vi "7HP_Get_serial_number.vi"(3 "timeout (ms)":u32=5000, 5 "Port":refnum<visa-resource-name>) -> (0 "Error Out":errorcluster, 2 "Serial number":u32)   [LabVIEW 2020]
uses:
  ctls/7HP_Cmd (USB).ctl
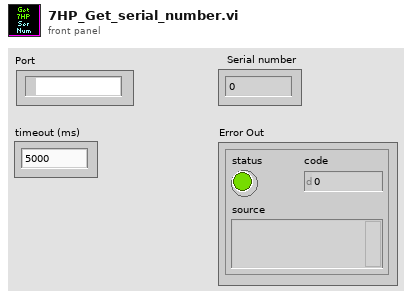
[diagram p1: front panel]
types:
  T1 = typedef "7HP_Cmd (USB).ctl" = string
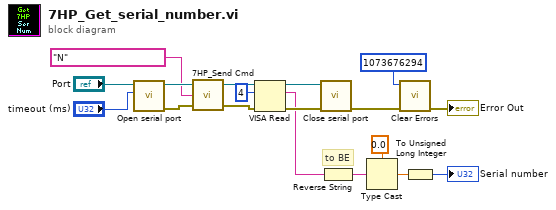
[diagram p0: block diagram]
diagram:
  # "to BE"
  n1 = call "Open serial port.vi"("timeout (ms)"="timeout (ms)", "VISA resource name"="Port") -> ("Error out"=w17:errorcluster, "VISA resource name out"=w18:refnum<visa-resource-name>)  [unwired: 8 in]
  n2 = call "7HP_Send Cmd.vi"("Error In"=w17, "Operation"=T1 "N", "Port"=w18) -> ("Error Out"=w15:errorcluster, "Port out"=w16:refnum<visa-resource-name>)  [unwired: 1 in]
  n3 = VISA Read(VISA resource name=w16, byte count=u32 4, error in (no error)=w15) -> (VISA resource name out=w13:refnum<visa-resource-name>, read buffer=w9:string, error out=w12:errorcluster)  [unwired: 1 out]
  n4 = call "Close serial port.vi"("Error in"=w12, "VISA resource name"=w13) -> ("Error out"=w4:errorcluster)  [unwired: 9 in]
  n5 = Reverse String(1:w9) -> (0:w10:string)
  n6 = Type Cast(type=sgl 0.0 ("byte count"), x=w10) -> (*(type *) &x=w8:sgl)
  n7 = call <vilib>:"Clear Errors.vi"("error in (no error)"=w4, "specific error code to clear (0: all)"=1073676294) -> ("error out"=→"Error Out":errorcluster)  [unwired: 4 in, 1 out]
  n8 = To Unsigned Long Integer(number=w8) -> (unsigned 32bit integer=→"Serial number":u32)
